vi "Robot Main.vi"() -> ()   [LabVIEW 2011]
doc: "This VI imlements the framework and scheduler for your robotics program. It should not be necessary to modify the framework. You are expected to add your code to the VIs called from Robot Main, the ones located in the Team Code within the project."
uses:
  <vilib>/Utility/RT CPU Load.ctl
  <vilib>/NI_Real-Time Target Support.lvlib
panel:
  out "Timings":cluster{"Call Name":string, "Delta (ms)":u32}[](array[cluster])
  out "CPU loads":T1[](array[typedef]) {"ISR (%)" format="%#.2f"; "Idle (%)" format="%#.2f"; "Background (%)" format="%#.2f"; "Normal (%)" format="%#.2f"; "Above Normal (%)" format="%#.2f"; "High (%)" format="%#.2g"; "Timed Structures (%)" format="%#.2g"; "Time Critical (%)" format="%#.2g"; "Total (%)" format="%#.2g"}
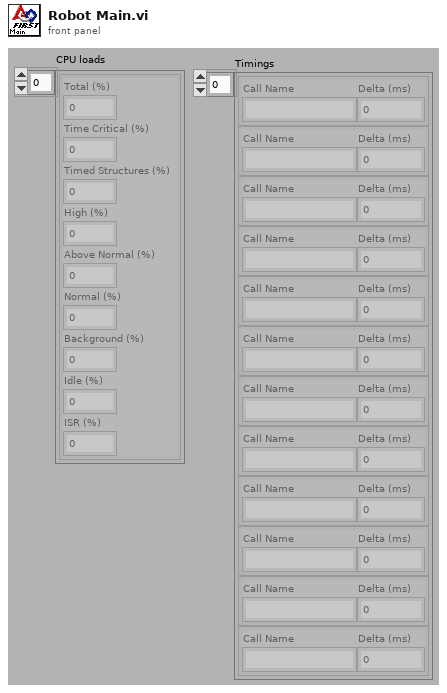
[diagram p1: front panel]
types:
  T1 = typedef "NI_Real-Time Target Support.lvlib/RT CPU Load.ctl" = cluster{"Total (%)":dbl, "Time Critical (%)":dbl, "Timed Structures (%)":dbl, "High (%)":dbl, "Above Normal (%)":dbl, "Normal (%)":dbl, "Background (%)":dbl, "Idle (%)":dbl, "ISR (%)":dbl}
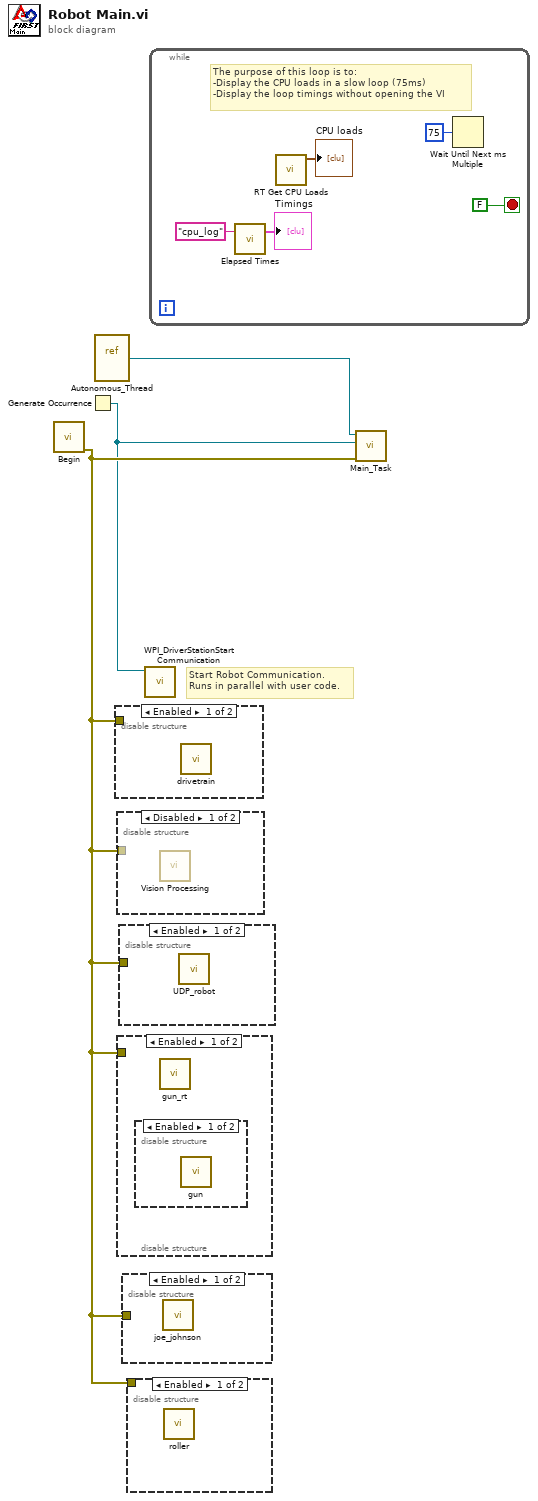
[diagram p0: block diagram]
diagram:
  # "Start Robot Communication.\nRuns in parallel with user code."
  n1 = call "Begin.vi"() -> ("error out"=w2:errorcluster)  [unwired: 1 in, 10 out]
  n2 = Generate Occurrence() -> (w1:refnum<k4>)
  n3 = vi-ref "Autonomous_Thread.vi"() -> (w3:refnum<vi>)
  n4 = disable-structure shown="Enabled" {
    disable-tunnel: w2 -> [_ _]
    frame Enabled {
      n5 = call "drivetrain.vi"() -> ()  [unwired: 12 in]
    }
    frame Disabled {
    }
  }
  n6 = disable-structure shown="Disabled" {
    disable-tunnel: w2 -> [_ _]
    frame Disabled {
      n7 = call "Vision Processing.vi"() -> ()  [unwired: 8 in]
    }
    frame Enabled {
    }
  }
  n8 = disable-structure shown="Enabled" {
    disable-tunnel: w2 -> [_ _]
    frame Enabled {
      n9 = disable-structure shown="Enabled" {
        frame Enabled {
          n10 = call "gun.vi"() -> ()  [unwired: 12 in]
        }
        frame Disabled {
        }
      }
      n11 = call "gun_rt.vi"() -> ()  [unwired: 12 in]
    }
    frame Disabled {
    }
  }
  n12 = disable-structure shown="Enabled" {
    disable-tunnel: w2 -> [_ _]
    frame Enabled {
      n13 = call "UDP_robot.vi"() -> ()  [unwired: 12 in]
    }
    frame Disabled {
    }
  }
  n14 = disable-structure shown="Enabled" {
    disable-tunnel: w2 -> [_ _]
    frame Enabled {
      n15 = call "joe_johnson.vi"() -> ()  [unwired: 12 in]
    }
    frame Disabled {
    }
  }
  n16 = disable-structure shown="Enabled" {
    disable-tunnel: w2 -> [_ _]
    frame Enabled {
      n17 = call "roller.vi"() -> ()  [unwired: 12 in]
    }
    frame Disabled {
    }
  }
  n18 = call <vilib>:"WPI_DriverStationStart Communication.vi"("occurrence"=w1) -> ()  [unwired: 11 out]
  n19 = while {
    stop <- FALSE stop-if-true
    # "The purpose of this loop is to:\n-Display the CPU loads in a slow loop (75ms)\n-Display the loop timings without opening the VI"
    n20 = call "Elapsed Times.vi"("Call Name"="cpu_log") -> ("Timings"=→"Timings":cluster{"Call Name":string, "Delta (ms)":u32}[])  [unwired: 2 in]
    n21 = call <vilib>:"RT Get CPU Loads.vi"() -> ("CPU loads"=→"CPU loads":T1[])  [unwired: 10 in, 1 out]
    n22 = Wait Until Next ms Multiple(millisecond multiple=u32 75) -> ()  [unwired: 1 out]
  }
  n23 = call "Main_Task.vi"("error in (no error)"=w2, "DS Occurence"=w1, "Autonomous VI in"=w3) -> ()  [unwired: 9 in]
